vi "ball management vi management.vi"(0 "Enum":enum16{"Init", "Run", "End"}(ring), 1 "De-Jam":bool, 5 "Bottom Front Sensor":bool, 7 "Bottom Back Sensor":bool, 9 "Shoot?":bool, 11 "# of Balls":dbl format="%#_1g") -> ()   [LabVIEW 2011]
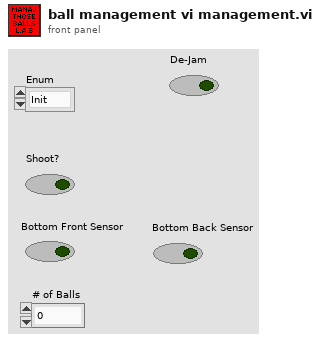
[diagram p1: front panel]
types:
  T1 = enum16{"Init", "Stop", "Convey", "Soft Convey", "DeJam", "End"}
  T2 = enum16{"Init", "Stop", "Shoot", "Reverse", "End"}
  T3 = enum16{"Init", "Stop", "Collect", "Slow Collect", "Reject", "End"}
  T4 = enum16{"Init", "Stop", "Collect", "Reject", "End"}
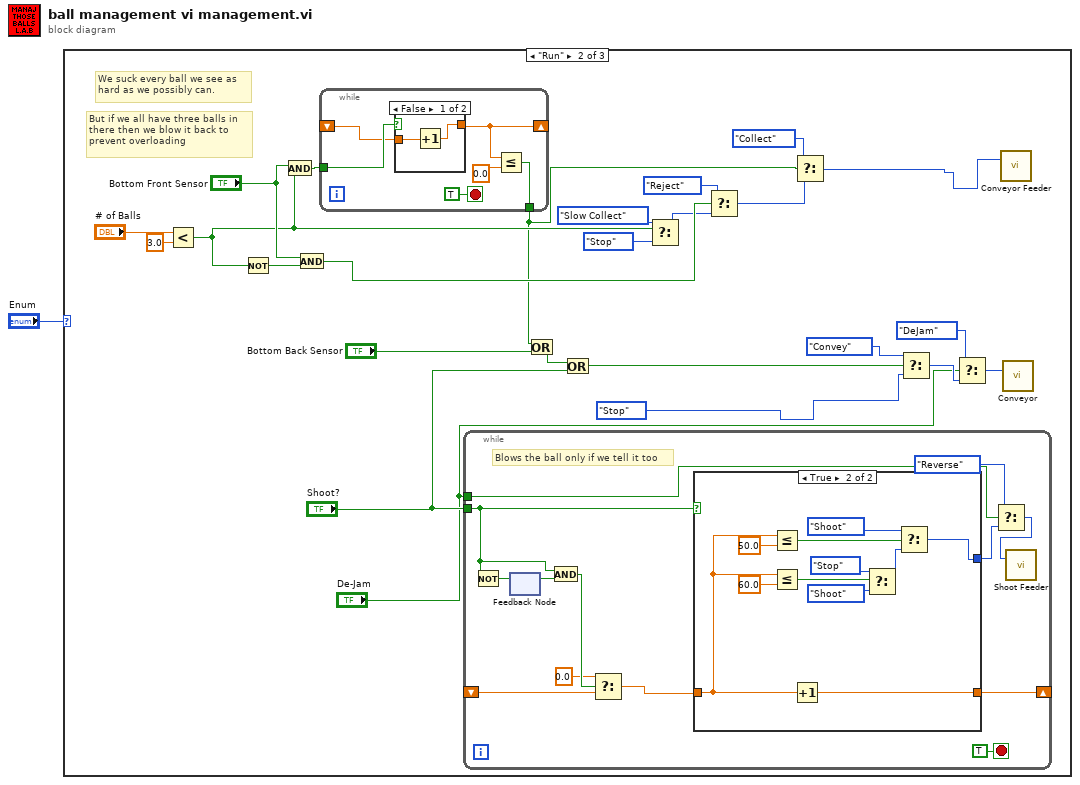
[diagram p0: block diagram]
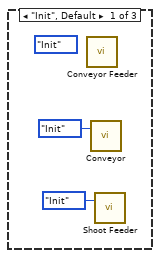
[diagram p2: hidden frame]
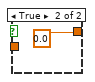
[diagram p3: hidden frame]
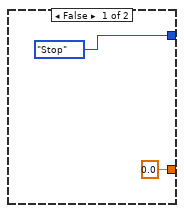
[diagram p4: hidden frame]
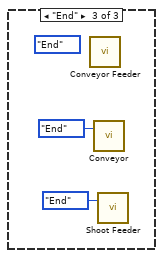
[diagram p5: hidden frame]
diagram:
  n1 = case shown="\"Run\"" "Enum" {
    frame "Init", Default {
      (unwired) T4."Init" ("Enum")
      n2 = call "Conveyor Feeder.vi"() -> ()  [unwired: 3 in]
      n3 = call "Conveyor.vi"("Enum"=T1."Init") -> ()  [unwired: 2 in]
      n4 = call "Shoot Feeder.vi"("Enum"=T2."Init") -> ()  [unwired: 2 in]
    }
    frame "Run" {
      # "But if we all have three balls in \nthere then we blow it back to \nprevent overloading"
      # "We suck every ball we see as \nhard as we possibly can."
      n5 = Less?(x="# of Balls", y=3.0) -> (x < y?=w15:bool)
      n6 = Not(x=w15) -> (.not. x?=w23:bool)
      n7 = And(x="Bottom Front Sensor", y=w15) -> (x .and. y?=w25:bool)
      n8 = And(x="Bottom Front Sensor", y=w23) -> (x .and. y?=w18:bool)
      n9 = while {
        shift-right: [w31] -> _
        shift-left: _ -> [w33]
        tunnel: w25 -> [w34]
        tunnel: [w29] -> w6
        stop <- TRUE stop-if-true
        n10 = case shown="False" w34 {
          tunnel: [w35 0.0] -> w31
          tunnel: w33 -> [w36 _]
          frame False {
            n11 = Increment(x=w36) -> (x+1=w35:dbl)
          }
          frame True {
          }
        }
        n12 = Less Or Equal?(x=w31, y=0.0) -> (x <= y?=w29:bool)
      }
      n13 = while {
        tunnel: "Shoot?" -> [w42]
        shift-right: [w44] -> _
        shift-left: _ -> [w46]
        tunnel: "De-Jam" -> [w41]
        stop <- TRUE stop-if-true
        # "Blows the ball only if we tell it too"
        n14 = Not(x=w42) -> (.not. x?=w50:bool)
        n15 = feedback #1() -> (w43:bool)  [unwired: 1 in]
        n16 = feedback-in #1(w50) -> ()
        n17 = And(x=w42, y=w43) -> (x .and. y?=w48:bool)
        n18 = Select(t=0.0, s=w48, f=w46) -> (s? t:f=w45:dbl)
        n19 = case shown="True" w42 {
          tunnel: w45 -> [_ w60]
          tunnel: [0.0 w63] -> w44
          tunnel: [T2."Stop" ("Enum") w53] -> w40
          frame False {
          }
          frame True {
            n20 = Less Or Equal?(x=w60, y=50.0) -> (x <= y?=w61:bool)
            n21 = Less Or Equal?(x=w60, y=60.0) -> (x <= y?=w58:bool)
            n22 = Increment(x=w60) -> (x+1=w63:dbl)
            n23 = Select(t=T2."Stop" ("Enum"), s=w58, f=T2."Shoot" ("Enum")) -> (s? t:f=w57:T2)
            n24 = Select(t=T2."Shoot" ("Enum"), s=w61, f=w57) -> (s? t:f=w53:T2)
          }
        }
        n25 = Select(t=T2."Reverse", s=w41, f=w40) -> (s? t:f=w38:T2)
        n26 = call "Shoot Feeder.vi"("Enum"=w38) -> ()  [unwired: 2 in]
      }
      n27 = Or(x=w6, y="Bottom Back Sensor") -> (x .or. y?=w21:bool)
      n28 = Or(x=w21, y="Shoot?") -> (x .or. y?=w26:bool)
      n29 = Select(t=T3."Slow Collect" ("Enum"), s=w15, f=T3."Stop" ("Enum")) -> (s? t:f=w12:T3)
      n30 = Select(t=T3."Reject" ("Enum"), s=w18, f=w12) -> (s? t:f=w19:T3)
      n31 = Select(t=T3."Collect" ("Enum"), s=w6, f=w19) -> (s? t:f=w4:T3)
      n32 = Select(t=T1."Convey" ("Enum"), s=w26, f=T1."Stop" ("Enum")) -> (s? t:f=w10:T1)
      n33 = Select(t=T1."DeJam" ("Enum"), s="De-Jam", f=w10) -> (s? t:f=w8:T1)
      n34 = call "Conveyor Feeder.vi"("Enum"=w4) -> ()  [unwired: 2 in]
      n35 = call "Conveyor.vi"("Enum"=w8) -> ()  [unwired: 2 in]
    }
    frame "End" {
      (unwired) T4."End" ("Enum")
      n36 = call "Conveyor Feeder.vi"() -> ()  [unwired: 3 in]
      n37 = call "Conveyor.vi"("Enum"=T1."End") -> ()  [unwired: 2 in]
      n38 = call "Shoot Feeder.vi"("Enum"=T2."End") -> ()  [unwired: 2 in]
    }
  }
